vi "getAttributeTreeUnitTooltip_action.vi"(0 "HGF_ImaqDx":refnum<class "HGF_ImaqDx.lvclass">, 1 "Tree Control In":refnum<vi>, 2 "Force update?":bool, 3 "Tab Control Ref In":T1, 5 "error in (no error)":errorcluster) -> (14 "dup HGF_ImaqDx":refnum<class "HGF_ImaqDx.lvclass">, 15 "Tree Control Out":refnum<vi>, 16 "Units":string, 17 "Tooltip":string, 19 "error out":errorcluster)   [LabVIEW 2014, in "HGF_IMAQ.lvlib" / "HGF_ImaqDx.lvclass"]
doc: "This is the override VI to read cameras attribute unit and tooltip."
uses:
  HGF_ImaqDx.lvclass
  HGF_VisionTools/HGF_VisionTools.lvlib
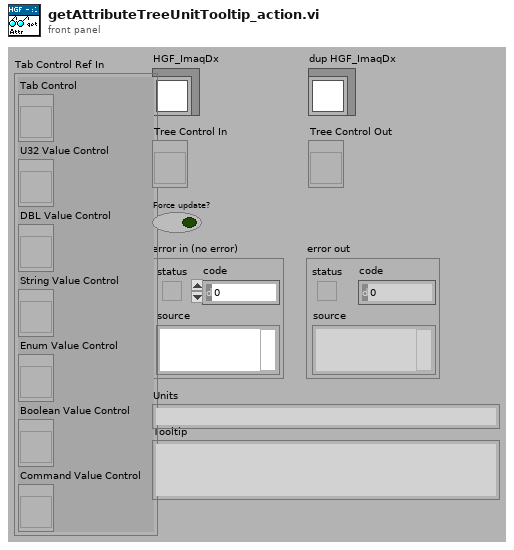
[diagram p1: front panel]
types:
  T1 = cluster{"Tab Control":refnum<vi>, "U32 Value Control":refnum<vi>, "DBL Value Control":refnum<vi>, "String Value Control":refnum<vi>, "Enum Value Control":refnum<vi>, "Boolean Value Control":refnum<vi>, "Command Value Control":refnum<vi>}
  T2 = typedef "IMAQdx.ctl" = refnum<k21>
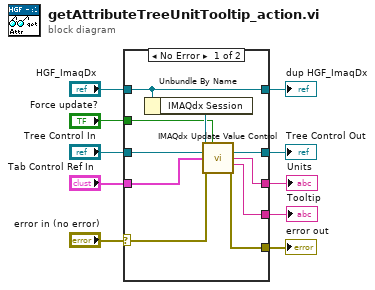
[diagram p0: block diagram]
diagram:
  n1 = case shown="No Error" "error in (no error)" {
    selector: "error in (no error)" -> [w16 w22]
    tunnel: [w18 w23] -> w9
    tunnel: "HGF_ImaqDx" -> [w18 w23]
    tunnel: [w15 w22] -> w7
    tunnel: [w19 w21] -> w6
    tunnel: "Tree Control In" -> [w20 w21]
    tunnel: "Tab Control Ref In" -> [w14 _]
    tunnel: "Force update?" -> [w13 _]
    tunnel: [w12 _] -> w2
    tunnel: [w11 _] -> w1
    frame No Error {
      n2 = Unbundle By Name(w18) -> ("IMAQdx Session"=w17:T2)
      n3 = call "IMAQdx Update Value Control.vi"("Session In"=w17, "Force update?"=w13, "Tree Control In"=w20, "Tab Control Ref In"=w14, "error in (no error)"=w16) -> ("Tree Control Out"=w19:refnum<vi>, "Units"=w12:string, "Tooltip"=w11:string, "error out"=w15:errorcluster)  [unwired: 6 in, 1 out]
    }
    frame Error {
    }
  }
  "error out" <- w7
  "dup HGF_ImaqDx" <- w9
  "Tree Control Out" <- w6
  "Units" <- w2
  "Tooltip" <- w1
